vi "Solar_V4_backup.vi"() -> ()   [LabVIEW 2012]
uses:
  <vilib>/Utility/file.llb/Write To Spreadsheet File (string).vi
panel:
  out "Wind Angle":sgl(knob) scale=0.0..360.0
  out "Wind Speed Speed":i16(knob) scale=0.0..100.0
  out "?":string
  out "inside":dbl(slide) scale=-10.0..50.0
  out "outside":dbl(slide) scale=-10.0..50.0
  in  "EXIT":bool
  out "LED":bool
  in  "stop":bool
  out "Energy":dbl format="%#.3f"
  out "Power":dbl format="%#.3f"
  out "Current":dbl format="%#.3f"
  out "Voltage":dbl format="%#.3f"
  out "Energy":dbl format="%#.3f"
  out "Power":dbl format="%#.3f"
  out "Current":dbl format="%#.3f"
  out "Voltage":dbl format="%#.3f"
  out "Energy":dbl format="%#.3f"
  out "Power":dbl format="%#.3f"
  out "Current":dbl format="%#.3f"
  out "Voltage":dbl format="%#.3f"
  out "Energy":dbl format="%#.3f"
  out "Power":dbl format="%#.3f"
  out "Current":dbl format="%#.3f"
  out "Voltage":dbl format="%#.3f"
  out "Energy":dbl format="%#.3f"
  out "Power":dbl format="%#.3f"
  out "Current":dbl format="%#.3f"
  out "Voltage":dbl format="%#.3f"
  out "Energy":dbl format="%#.3f"
  out "Power":dbl format="%#.3f"
  out "Current":dbl format="%#.3f"
  out "Voltage":dbl format="%#.3f"
  out "Energy":dbl format="%#.3f"
  out "Power":dbl format="%#.3f"
  out "Current":dbl format="%#.3f"
  out "Voltage":dbl format="%#.3f"
  out "Poly Si 1":dbl=1.3668
  out "Poly Si 2":dbl=1.3668
  out "Thin film 2":dbl=1.3668
  out "thin Film 1":dbl=1.3668
  out "DSSC3":dbl=1.0
  out "DSSC 2":dbl=0.01296
  out "DSSC 1":dbl=0.375
  out "Waveform Chart":dynamicdata(graph)
  in  "Solar Related":T1(tab)
  out "Solar Tilted":dynamicdata(graph)
  out "Solar vertical":dynamicdata(graph)
  out "Solar Tracked":dynamicdata(graph)
  out "Solar Meteo":dynamicdata(graph)
  out "Solar UV":dynamicdata(graph)
  in  "TEMPERATURES":T2(tab)
  out "Temperature DSSC 1":dynamicdata(graph)
  out "Temperature DSSC 2":dynamicdata(graph)
  out "Temperature Poly Si":dynamicdata(graph)
  out "Temperature Thin Film":dynamicdata(graph)
  out "Array":dbl[][](array[numeric])
  # "DSSC 1"
  # "DSSC 2"
  # "DSSC 3"
  # "Poly Si 1"
  # "Poly Si 2"
  # "Thin Film 1"
  # "Thin Film 2"
  # "Temperatures"
  # "Weather Station"
  # "DSSC 1"
  # "DSSC 2"
  # "DSSC 3"
  # "Poly Si 1"
  # "Poly Si  2"
  # "Thin Film 1"
  # "Thin Film 2"
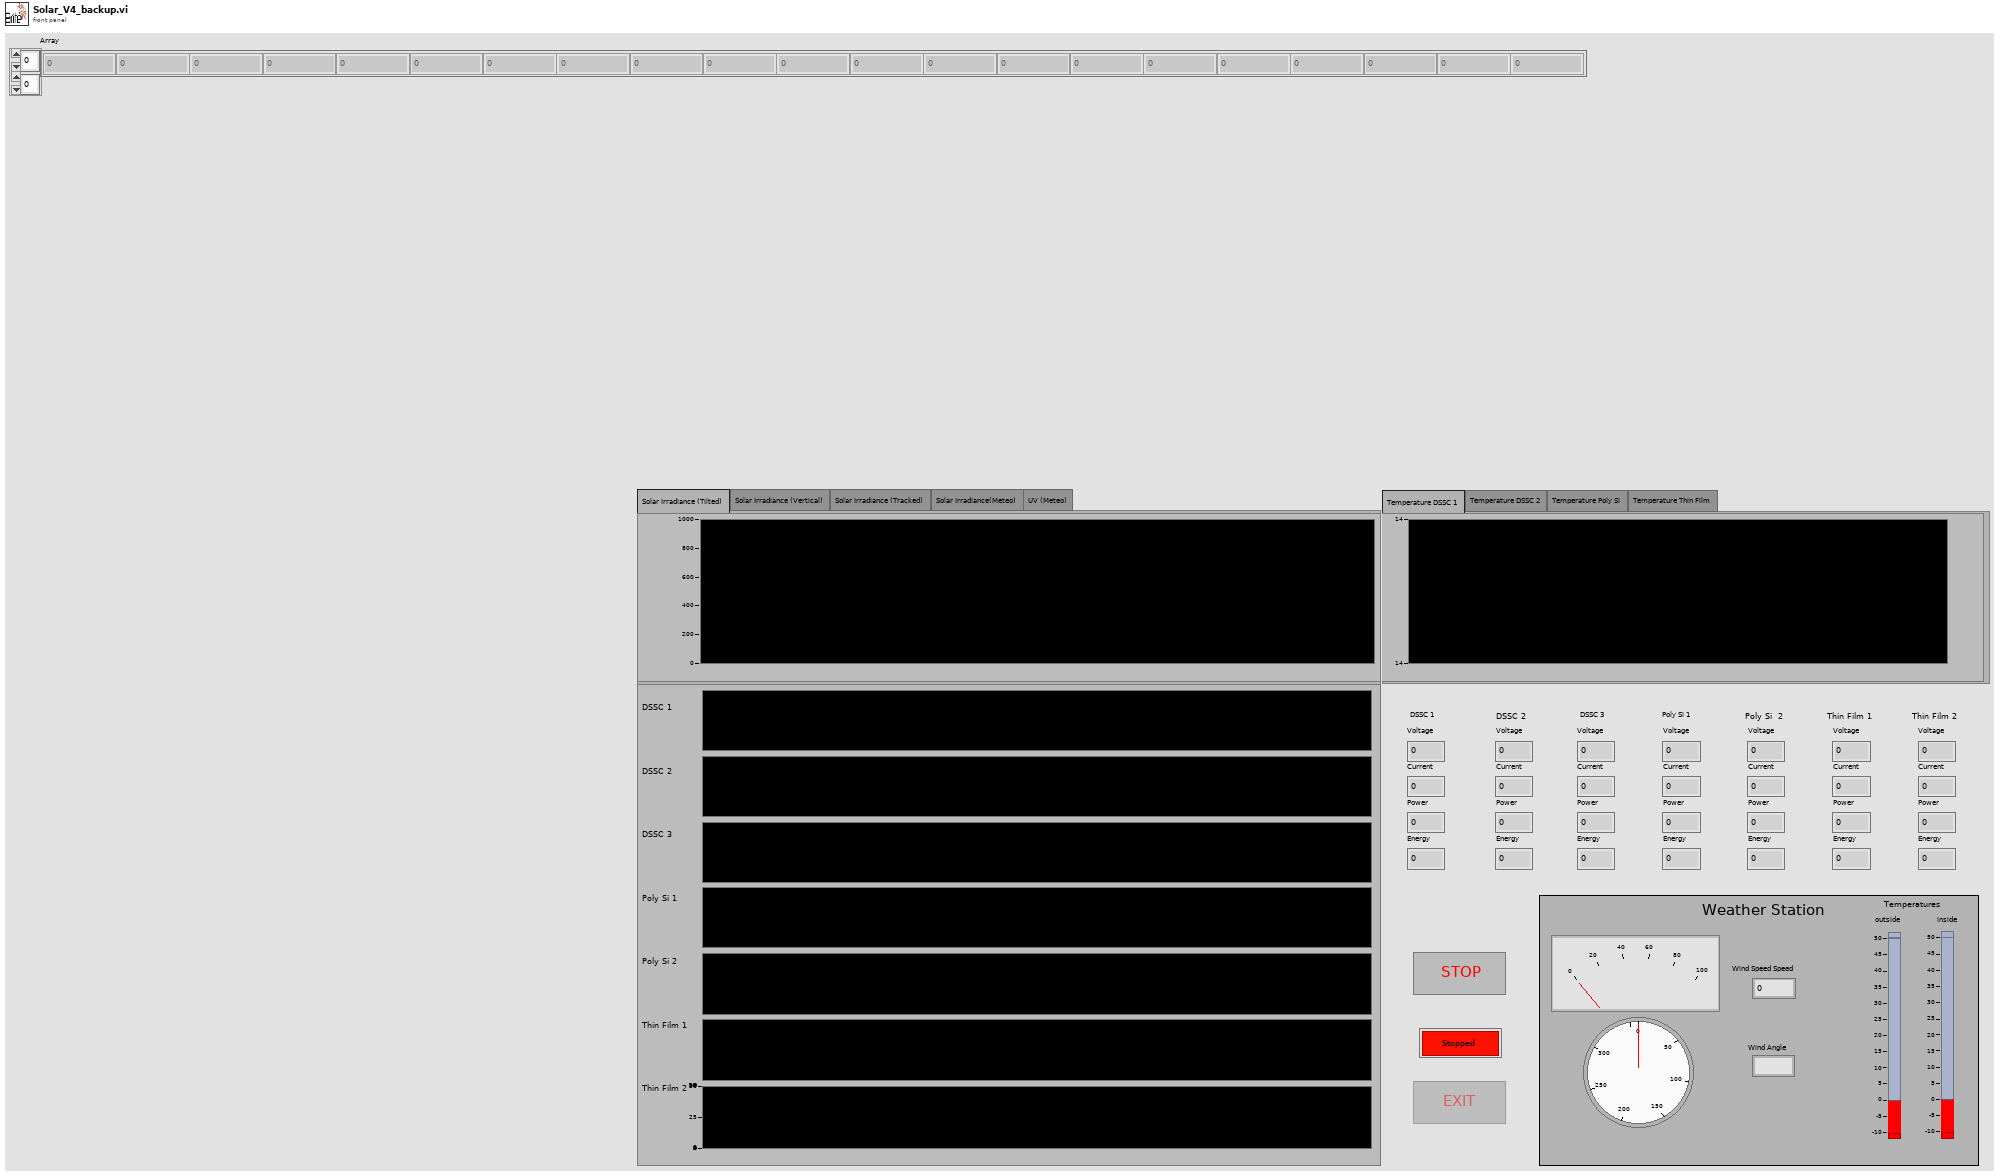
[diagram p1: front panel]
types:
  T1 = enum32{"Solar Irradiance (Tilted)", "Solar Irradiance (Vertical)", "Solar Irradiance (Tracked)", "Solar Irradiance(Meteo)", "UV (Meteo)"}
  T2 = enum32{"Temperature DSSC 1", "Temperature DSSC 2", "Temperature Poly Si", "Temperature Thin Film"}
  T3 = enum8{"Enabled", "Disabled", "Disabled and Grayed Out"}
  T4 = enum16{"open", "replace", "create", "open or create", "replace or create", "replace or create with confirmation"}
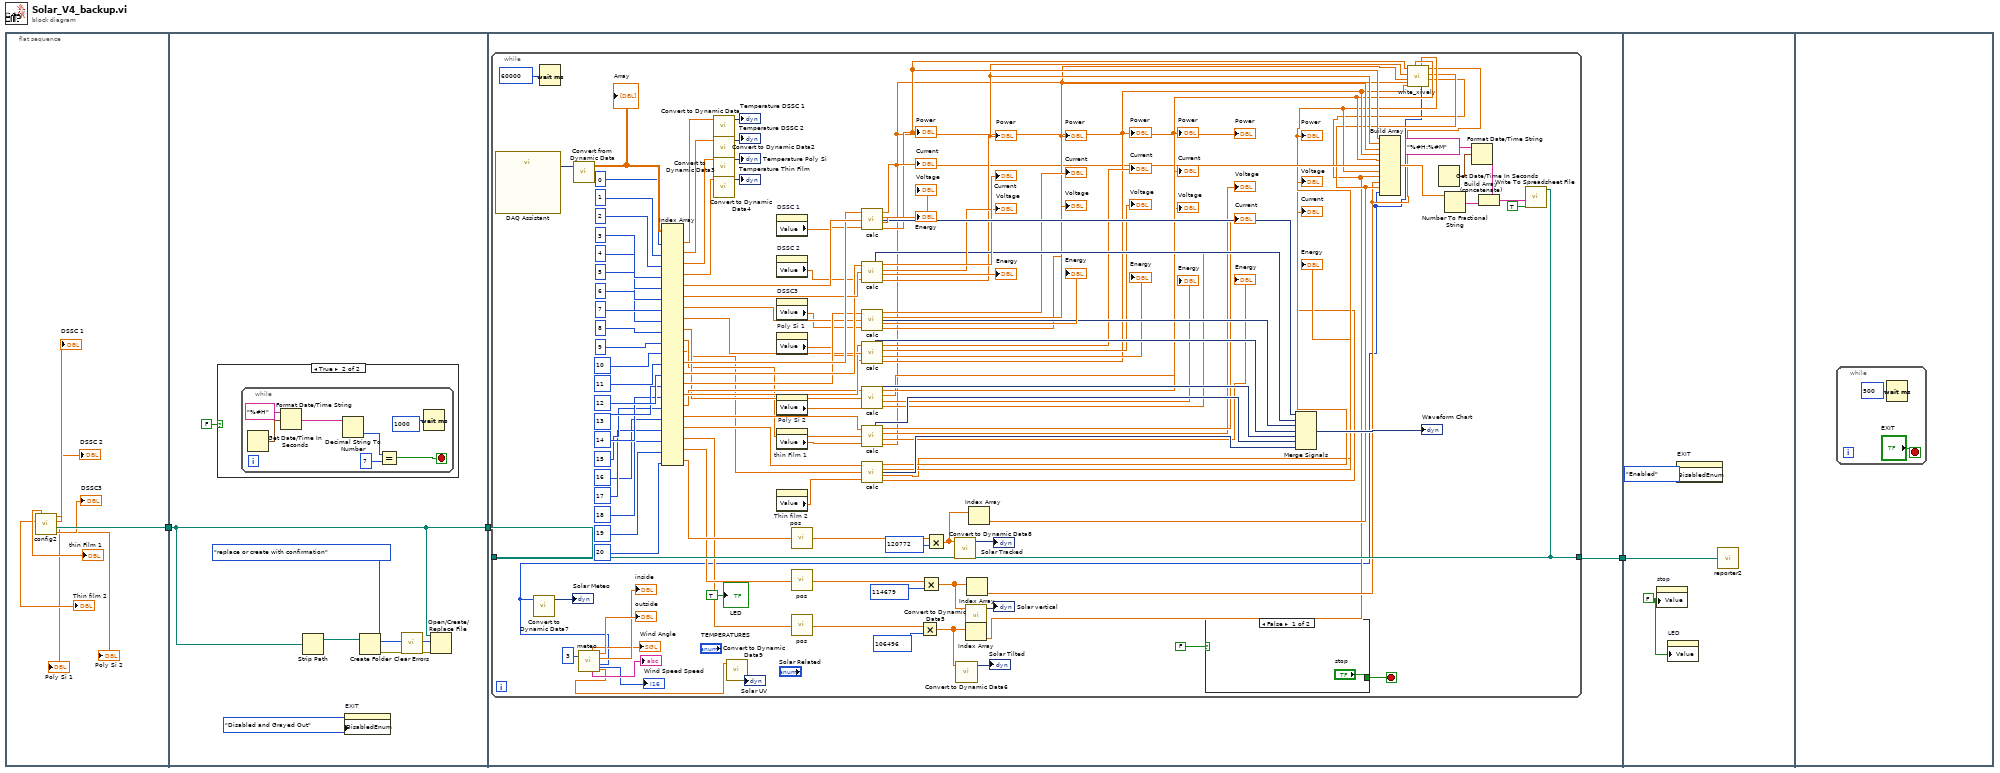
[diagram p0: block diagram]
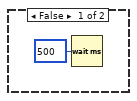
[diagram p2: hidden frame]
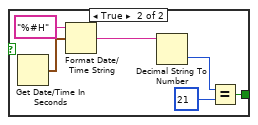
[diagram p3: hidden frame]
diagram:
  n1 = flat-sequence {
    tunnel: [w11] -> w3
    tunnel: w3 -> [w14]
    tunnel: [w14] -> w2
    tunnel: w2 -> [w28]
    tunnel: [w27] -> w1
    tunnel: w1 -> [w166]
    frame #0 {
      n2 = call "config2.vi"() -> ("DSSC3"=→"DSSC3":dbl, "path"=w11:path, "DSSC 1"=→"DSSC 1":dbl, "DSSC 2"=→"DSSC 2":dbl, "Poly Si 2"=→"Poly Si 2":dbl, "Poly Si 1"=→"Poly Si 1":dbl, "thin Film 2"=→"Thin film 2":dbl, "thin Film 1"=→"thin Film 1":dbl)
    }
    frame #1 {
      n3 = case shown="True" FALSE {
        frame False {
          n4 = Wait (ms)(milliseconds to wait=u32 500) -> ()  [unwired: 1 out]
        }
        frame True {
          n5 = while {
            stop <- w20 stop-if-true
            n6 = Get Date/Time In Seconds() -> (seconds since 1Jan1904=w26:timestamp)
            n7 = Format Date/Time String(time format string (%c)="%#H", seconds (now)=w26) -> (date/time string=w23:string)  [unwired: 1 in]
            n8 = Decimal String To Number(string=w23) -> (number=w22:i32)  [unwired: 2 in, 1 out]
            n9 = Equal?(x=w22, y=7) -> (x = y?=w20:bool)
            n10 = Wait (ms)(milliseconds to wait=u32 1000) -> ()  [unwired: 1 out]
          }
        }
      }
      n11 = Strip Path(path=w14) -> (stripped path=w17:path)  [unwired: 1 out]
      n12 = property on="EXIT" class="Bool"("DisabledEnum"=T3."Disabled and Grayed Out" ("Disabled")) -> ()  [unwired: 2 in, 2 out]
      n13 = Create Folder(path (use dialog)=w17) -> (error out=w16:errorcluster)  [unwired: 2 in, 2 out]
      n14 = call <vilib>:"Clear Errors.vi"("error in (no error)"=w16) -> ("error out"=w15:errorcluster)  [unwired: 6 in]
      n15 = Open/Create/Replace File(file path (use dialog)=w14, error in=w15, operation (0:open)=T4."replace or create with confirmation") -> ()  [unwired: 3 in, 3 out]
    }
    frame #2 {
      n16 = while {
        tunnel: w28 -> [w131]
        tunnel: [w131] -> w27
        stop <- w130 stop-if-true
        n17 = call "DAQ Assistant"() -> ("data"=w132:dynamicdata)  [unwired: 17 in, 2 out]
        n18 = Wait (ms)(milliseconds to wait=u32 60000) -> ()  [unwired: 1 out]
        n19 = call "Convert from Dynamic Data"("Dynamic Data Type"=w132) -> ("Array"=w156:dbl[][])  [unwired: 3 in]
        "Array" <- w156
        n20 = call "meteo.vi"("ComPort 2"=i16 3) -> ("Wind Speed 2"=→"Wind Speed Speed":i16, "Wind Angle 2"=→"Wind Angle":sgl, "Direction 2"=→"?":string, "Outside Temperature"=→"outside":sgl, "Inside Temp"=→"inside":sgl, "Solar"=w32:i16, "UV"=w29:sgl)
        n21 = call "Convert to Dynamic Data7"("Double"=w32) -> ("Dynamic Data Type"=→"Solar Meteo":dynamicdata)  [unwired: 3 in]
        n22 = Index Array(array=w156, index (col) #1=0 ("index (row)"), index (col) #2=1 ("index (col)"), index (col) #3=2 ("index (col)"), index (col) #4=3 ("index (col)"), index (col) #5=4 ("index (col)"), index (col) #6=5 ("index (col)"), index (col) #7=6 ("index (col)"), index (col) #8=7 ("index (col)"), index (col) #9=8 ("index (col)"), index (col) #10=9 ("index (col)"), index (col) #11=10 ("index (col)"), index (col) #12=11 ("index (col)"), index (col) #13=12 ("index (col)"), index (col) #14=13 ("index (col)"), index (col) #15=14 ("index (col)"), index (col) #16=15 ("index (col)"), index (col) #17=16 ("index (col)"), index (col) #18=17 ("index (col)"), index (col) #19=18 ("index (col)"), index (col) #20=19 ("index (col)"), index (col) #21=20 ("index (col)")) -> (element #1=w71:dbl[], element #2=w70:dbl[], element #3=w69:dbl[], element #4=w68:dbl[], element #5=w122:dbl[], element #6=w112:dbl[], element #7=w109:dbl[], element #8=w104:dbl[], element #9=w86:dbl[], element #10=w85:dbl[], element #11=w84:dbl[], element #12=w121:dbl[], element #13=w111:dbl[], element #14=w110:dbl[], element #15=w90:dbl[], element #16=w89:dbl[], element #17=w88:dbl[], element #18=w87:dbl[], element #19=w55:dbl[], element #20=w56:dbl[], element #21=w91:dbl[])  [unwired: 21 in]
        n23 = call "Convert to Dynamic Data"("Array"=w71) -> ("Dynamic Data Type"=→"Temperature DSSC 1":dynamicdata)  [unwired: 3 in]
        n24 = call "Convert to Dynamic Data2"("Array"=w70) -> ("Dynamic Data Type"=→"Temperature DSSC 2":dynamicdata)  [unwired: 3 in]
        n25 = call "Convert to Dynamic Data3"("Array"=w69) -> ("Dynamic Data Type"=→"Temperature Poly Si":dynamicdata)  [unwired: 3 in]
        n26 = call "Convert to Dynamic Data4"("Array"=w68) -> ("Dynamic Data Type"=→"Temperature Thin Film":dynamicdata)  [unwired: 3 in]
        n27 = call "Convert to Dynamic Data9"("Double"=w29) -> ("Dynamic Data Type"=→"Solar UV":dynamicdata)  [unwired: 3 in]
        n28 = property on="DSSC 1" class="DigNum (strict)"() -> ("Value"=w67:dbl)  [unwired: 2 in, 2 out]
        n29 = property on="DSSC 2" class="DigNum (strict)"() -> ("Value"=w66:dbl)  [unwired: 2 in, 2 out]
        n30 = property on="DSSC3" class="DigNum (strict)"() -> ("Value"=w65:dbl)  [unwired: 2 in, 2 out]
        n31 = property on="Poly Si 1" class="DigNum (strict)"() -> ("Value"=w62:dbl)  [unwired: 2 in, 2 out]
        n32 = property on="Poly Si 2" class="DigNum (strict)"() -> ("Value"=w61:dbl)  [unwired: 2 in, 2 out]
        n33 = property on="thin Film 1" class="DigNum (strict)"() -> ("Value"=w64:dbl)  [unwired: 2 in, 2 out]
        n34 = property on="Thin film 2" class="DigNum (strict)"() -> ("Value"=w63:dbl)  [unwired: 2 in, 2 out]
        n35 = call "pos.vi"("Input"=w91) -> ("Output"=w129:dbl[])
        n36 = call "pos.vi"("Input"=w56) -> ("Output"=w59:dbl[])
        n37 = call "pos.vi"("Input"=w55) -> ("Output"=w57:dbl[])
        n38 = call "calc.vi"("Input Current"=w121, "Input voltage"=w122, "Area factor"=w67) -> ("Current"=→"Current":dbl, "Voltage"=→"Voltage":dbl, "Energy"=→"Energy":dbl, "Power"=w42:dbl, "Waveform Chart"=w118:dynamicdata)
        "Power" <- w42
        n39 = call "calc.vi"("Input Current"=w111, "Input voltage"=w112, "Area factor"=w66) -> ("Current"=→"Current":dbl, "Voltage"=→"Voltage":dbl, "Energy"=→"Energy":dbl, "Power"=w41:dbl, "Waveform Chart"=w113:dynamicdata)
        "Power" <- w41
        n40 = call "calc.vi"("Input Current"=w110, "Input voltage"=w109, "Area factor"=w65) -> ("Current"=→"Current":dbl, "Voltage"=→"Voltage":dbl, "Energy"=→"Energy":dbl, "Power"=w40:dbl, "Waveform Chart"=w105:dynamicdata)
        "Power" <- w40
        n41 = call "calc.vi"("Input Current"=w90, "Input voltage"=w104, "Area factor"=w62) -> ("Current"=→"Current":dbl, "Voltage"=→"Voltage":dbl, "Energy"=→"Energy":dbl, "Power"=w39:dbl, "Waveform Chart"=w103:dynamicdata)
        "Power" <- w39
        n42 = call "calc.vi"("Input Current"=w89, "Input voltage"=w86, "Area factor"=w61) -> ("Current"=→"Current":dbl, "Voltage"=→"Voltage":dbl, "Energy"=→"Energy":dbl, "Power"=w38:dbl, "Waveform Chart"=w83:dynamicdata)
        "Power" <- w38
        n43 = call "calc.vi"("Input Current"=w88, "Input voltage"=w85, "Area factor"=w64) -> ("Current"=→"Current":dbl, "Voltage"=→"Voltage":dbl, "Energy"=→"Energy":dbl, "Power"=w37:dbl, "Waveform Chart"=w82:dynamicdata)
        "Power" <- w37
        n44 = call "calc.vi"("Input Current"=w87, "Input voltage"=w84, "Area factor"=w63) -> ("Current"=→"Current":dbl, "Voltage"=→"Voltage":dbl, "Energy"=→"Energy":dbl, "Power"=w36:dbl, "Waveform Chart"=w81:dynamicdata)
        "Power" <- w36
        n45 = Multiply(x=w57, y=106496) -> (x*y=w50:dbl[])
        n46 = Multiply(x=w59, y=114679) -> (x*y=w51:dbl[])
        n47 = Multiply(x=w129, y=120772) -> (x*y=w52:dbl[])
        n48 = call "Convert to Dynamic Data8"("Array"=w52) -> ("Dynamic Data Type"=→"Solar Tracked":dynamicdata)  [unwired: 3 in]
        n49 = call "Convert to Dynamic Data6"("Array"=w50) -> ("Dynamic Data Type"=→"Solar Tilted":dynamicdata)  [unwired: 3 in]
        n50 = call "Convert to Dynamic Data5"("Array"=w51) -> ("Dynamic Data Type"=→"Solar vertical":dynamicdata)  [unwired: 3 in]
        n51 = Index Array(array=w50) -> (element=w33:dbl)  [unwired: 1 in]
        n52 = Index Array(array=w51) -> (element=w34:dbl)  [unwired: 1 in]
        n53 = Index Array(array=w52) -> (element=w35:dbl)  [unwired: 1 in]
        n54 = case shown="False" FALSE {
          tunnel: ["stop" w158] -> w130
          frame False {
          }
          frame True {
            n55 = Get Date/Time In Seconds() -> (seconds since 1Jan1904=w163:timestamp)
            n56 = Format Date/Time String(time format string (%c)="%#H", seconds (now)=w163) -> (date/time string=w161:string)  [unwired: 1 in]
            n57 = Decimal String To Number(string=w161) -> (number=w160:i32)  [unwired: 2 in, 1 out]
            n58 = Equal?(x=w160, y=21) -> (x = y?=w158:bool)
          }
        }
        n59 = Merge Signals(w118, w113, w105, w103, w83, w82, w81) -> (→"Waveform Chart":dynamicdata)
        n60 = Build Array(w42, w41, w40, w39, w38, w37, w36, w33, w34, w35, w32) -> (w135:dbl[])
        n61 = call "write_xively.vi"("Solar__Tilted_"=w33, "Solar__Tracked_"=w35, "Solar__Vertical_"=w34, "Solar__meteo_"=w32, "Thin_Film_2"=w36, "Thin_Film_1"=w37, "Poly Si 2"=w38, "Poly Si 1"=w39, "DSSC3"=w40, "DSSC2"=w41, "DSSC1"=w42) -> ()  [unwired: 1 in]
        n62 = Get Date/Time In Seconds() -> (seconds since 1Jan1904=w139:timestamp)
        n63 = Number To Fractional String(number=w135) -> (F-format string=w136:string[])  [unwired: 3 in]
        n64 = Format Date/Time String(time format string (%c)="%#H:%#M", seconds (now)=w139) -> (date/time string=w137:string)  [unwired: 1 in]
        n65 = Build Array (concatenate)(w137, w136) -> (w134:string[])
        n66 = call-poly <vilib>:"Write To Spreadsheet File.vi"("append to file? (new file:F)"=TRUE, "1D data"=w134, "file path (dialog if empty)"=w131) -> ()  [unwired: 5 in, 1 out]
        "LED" <- TRUE
      }
    }
    frame #3 {
      w164 = FALSE ("stop")
      n67 = property on="stop" class="Bool (strict)"("Value"=w164) -> ()  [unwired: 2 in, 2 out]
      n68 = property on="LED" class="Bool (strict)"("Value"=w164) -> ()  [unwired: 2 in, 2 out]
      n69 = property on="EXIT" class="Bool"("DisabledEnum"=T3."Enabled" ("Disabled")) -> ()  [unwired: 2 in, 2 out]
      n70 = call "reporter2.vi"("file path (dialog if empty)"=w166) -> ()  [unwired: 1 out]
    }
    frame #4 {
      n71 = while {
        stop <- "EXIT" stop-if-true
        n72 = Wait (ms)(milliseconds to wait=u32 500) -> ()  [unwired: 1 out]
      }
    }
  }
